vi "Run.vi"(2 "D_Angle":dbl, 3 "Angle":dbl, 4 "Encoder":dbl) -> (0 "PWM":dbl)   [LabVIEW 2018]
uses:
  Global_variables.vi
panel:
  out "exp(x)":dbl
  in  "Flag_Back 2":dbl
  in  "Count_keep_balance":dbl
  in  "Count_P2":dbl
  in  "count_position":dbl
  in  "Position_Max":dbl
  in  "Angle_Max":dbl
  in  "Count_Big_Angle":dbl
  in  "Flag_Back":dbl
  in  "Target_position":dbl
  in  "Count_Next":dbl
  in  "Count_FZ":dbl
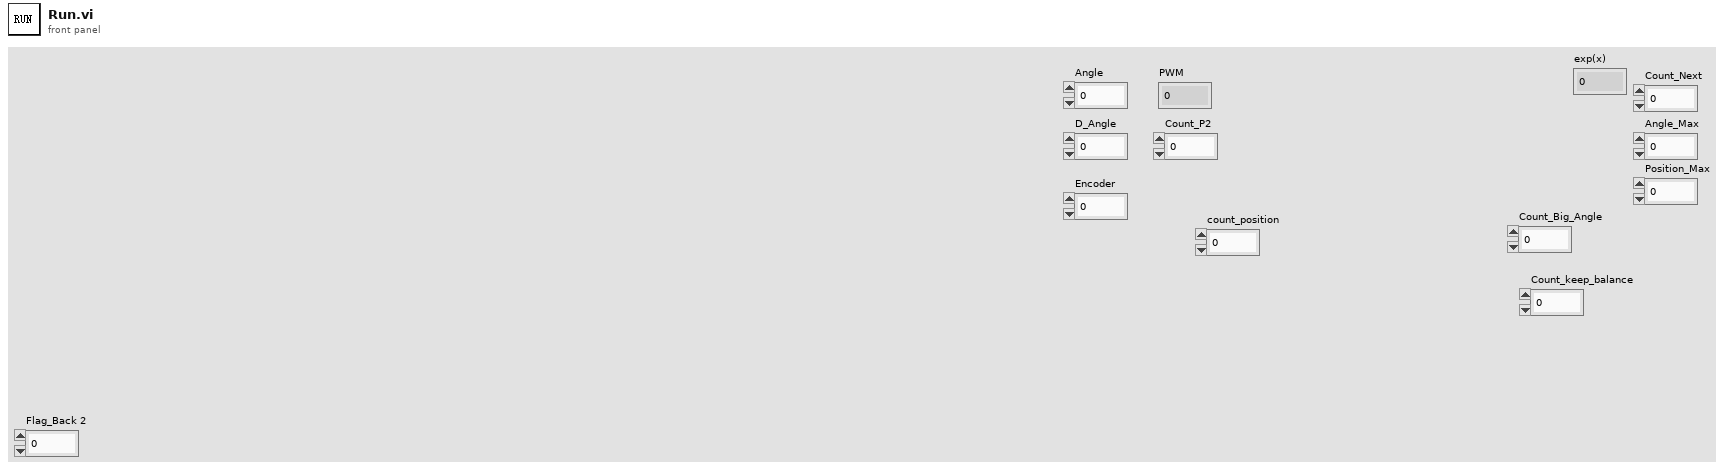
[diagram p1: front panel]
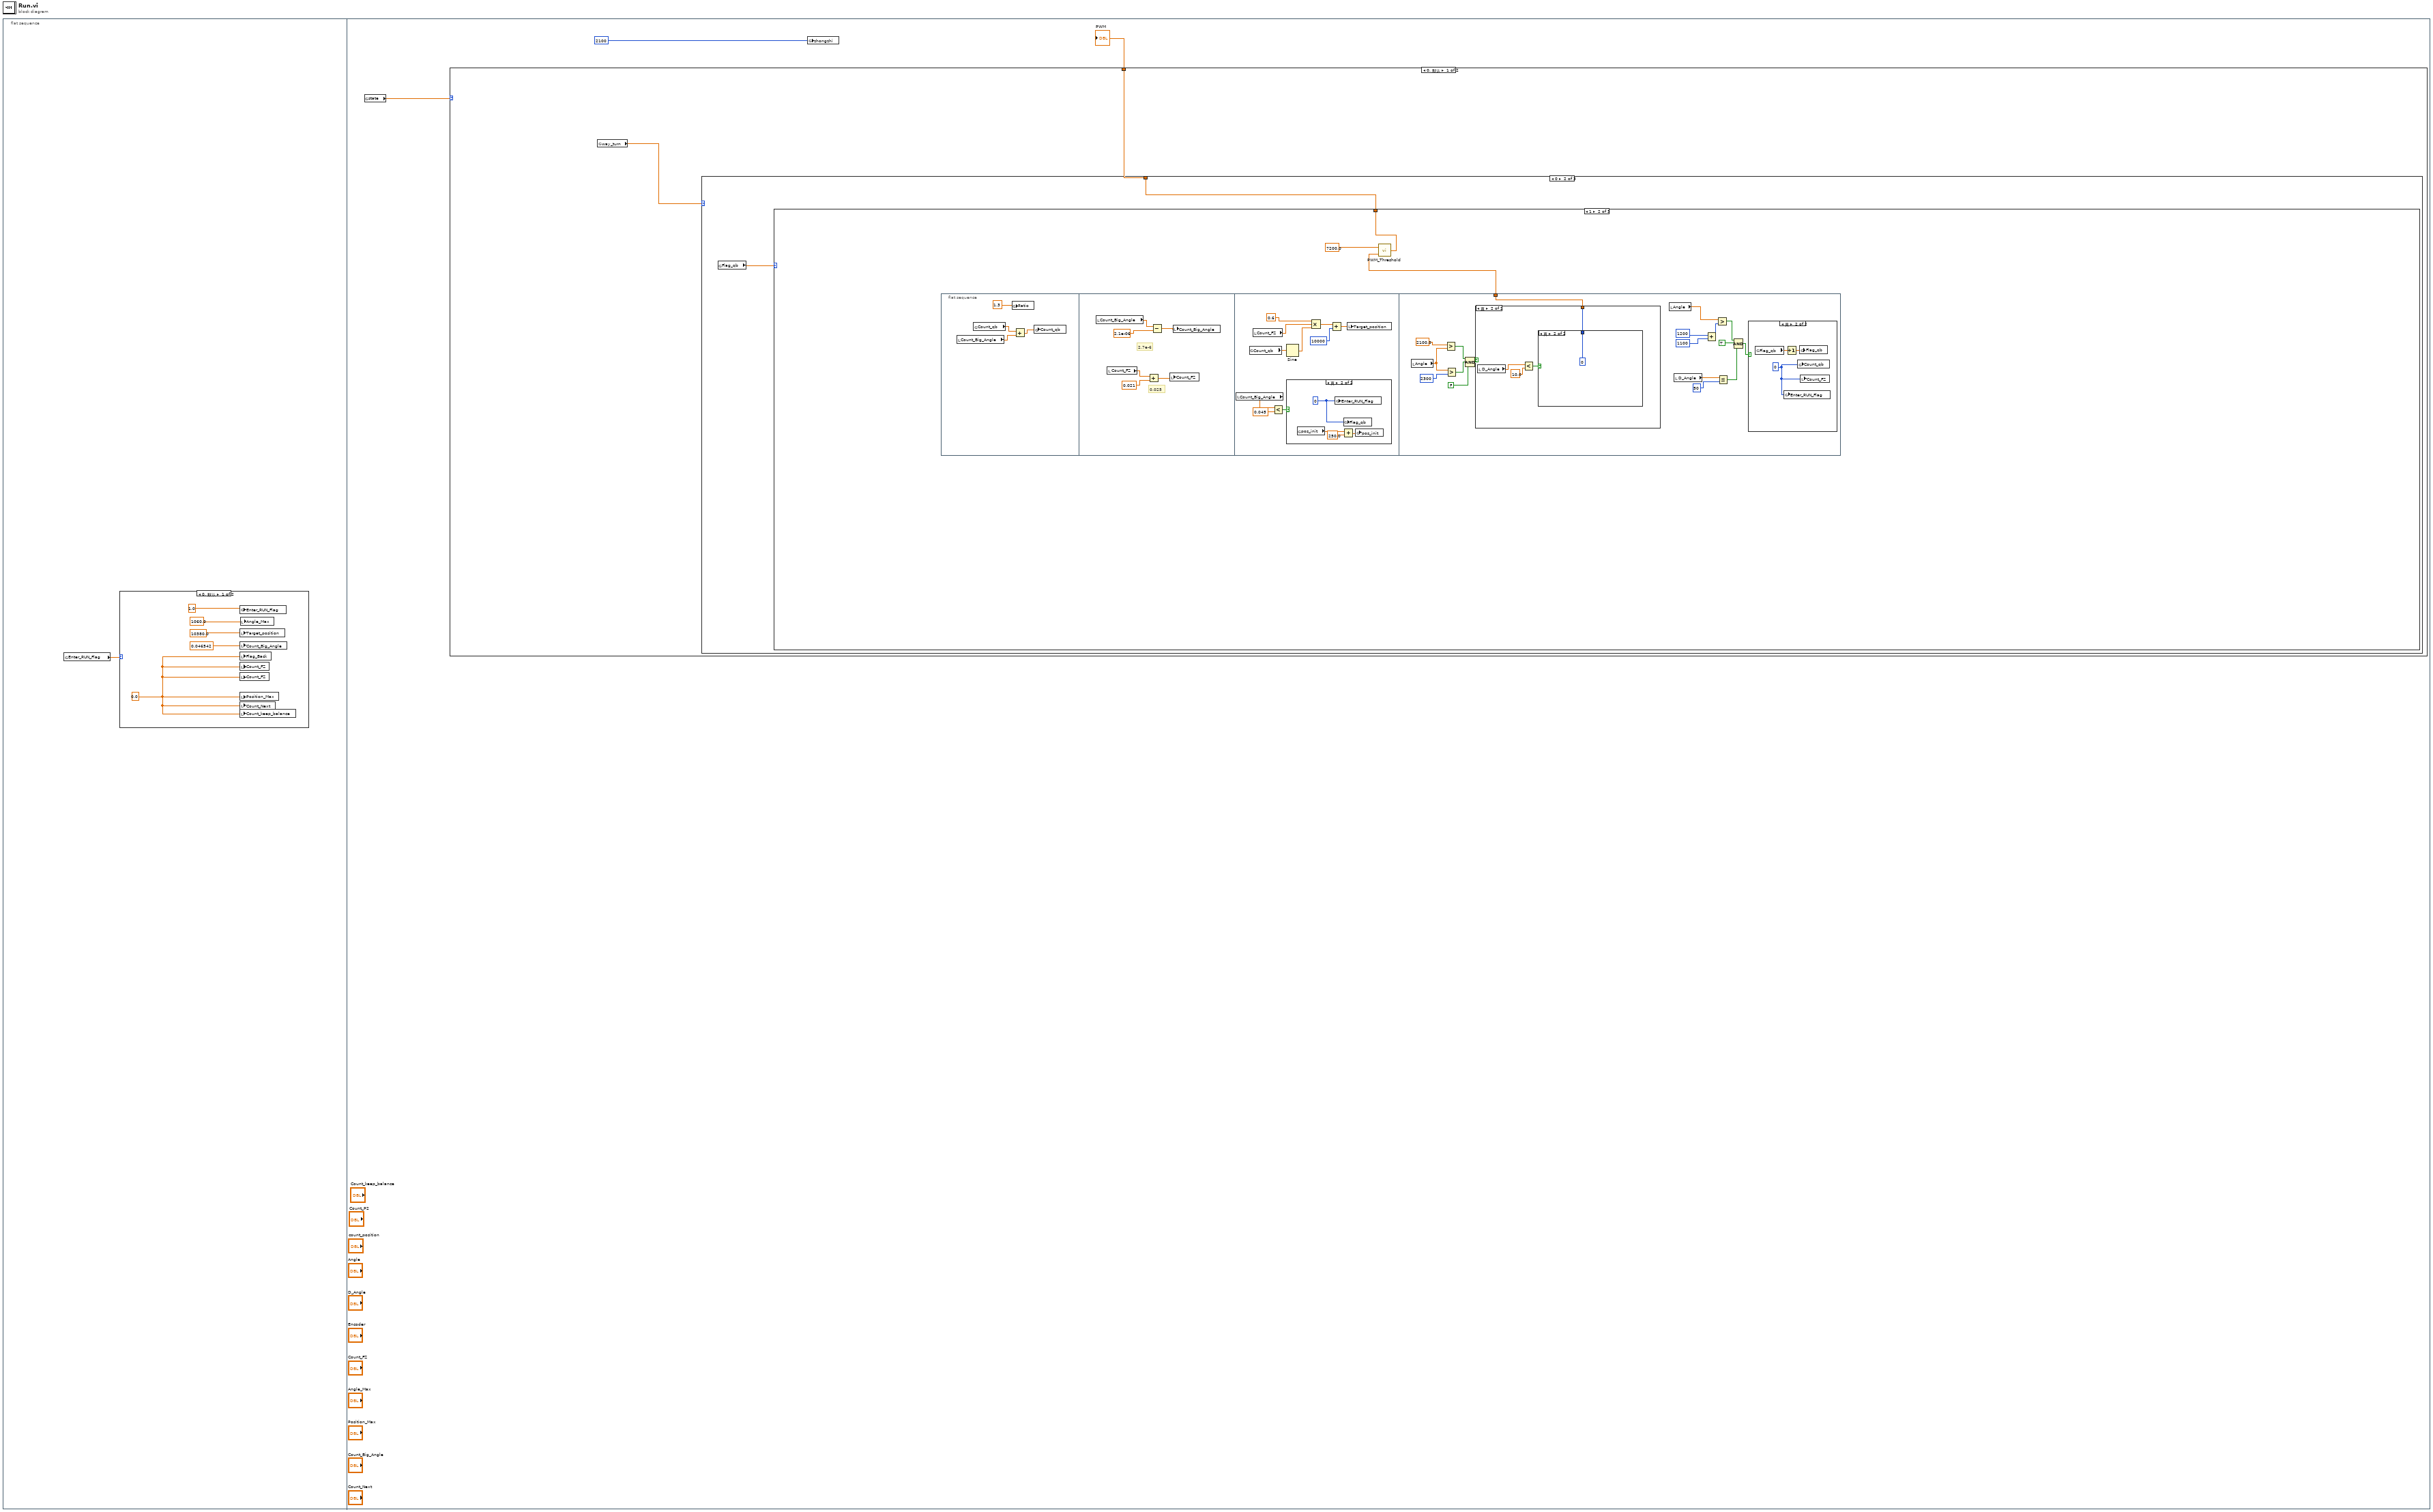
[diagram p0: block diagram]
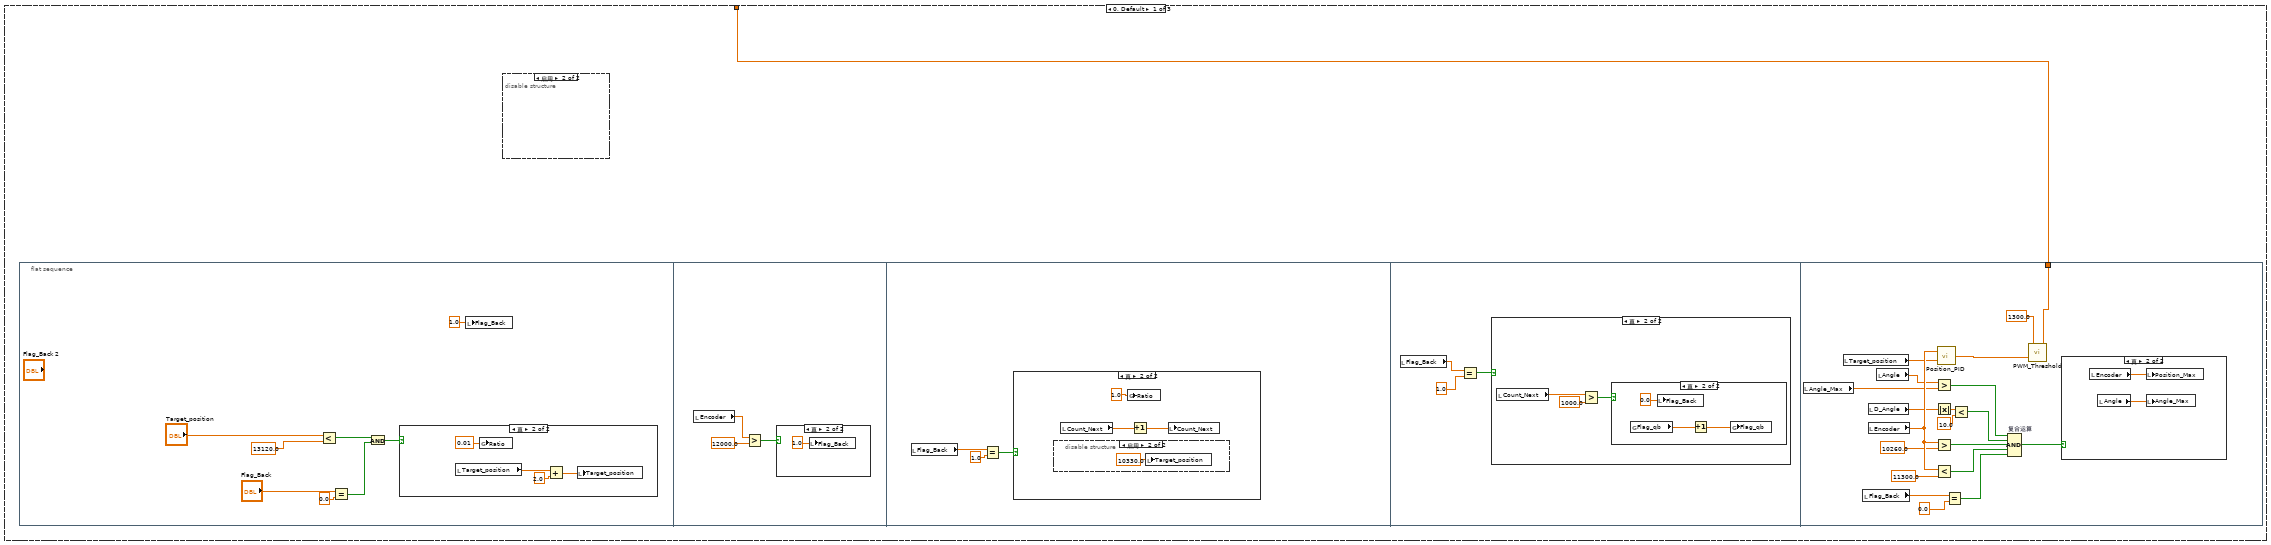
[diagram p4: hidden frame]
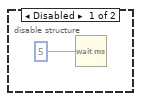
[diagram p5: hidden frame]
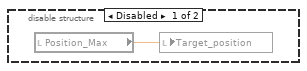
[diagram p9: hidden frame]
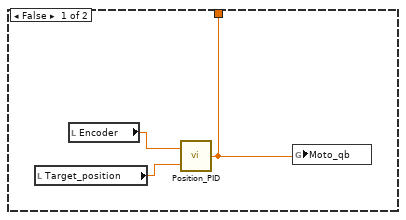
[diagram p14: hidden frame]
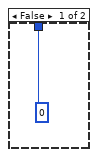
[diagram p15: hidden frame]
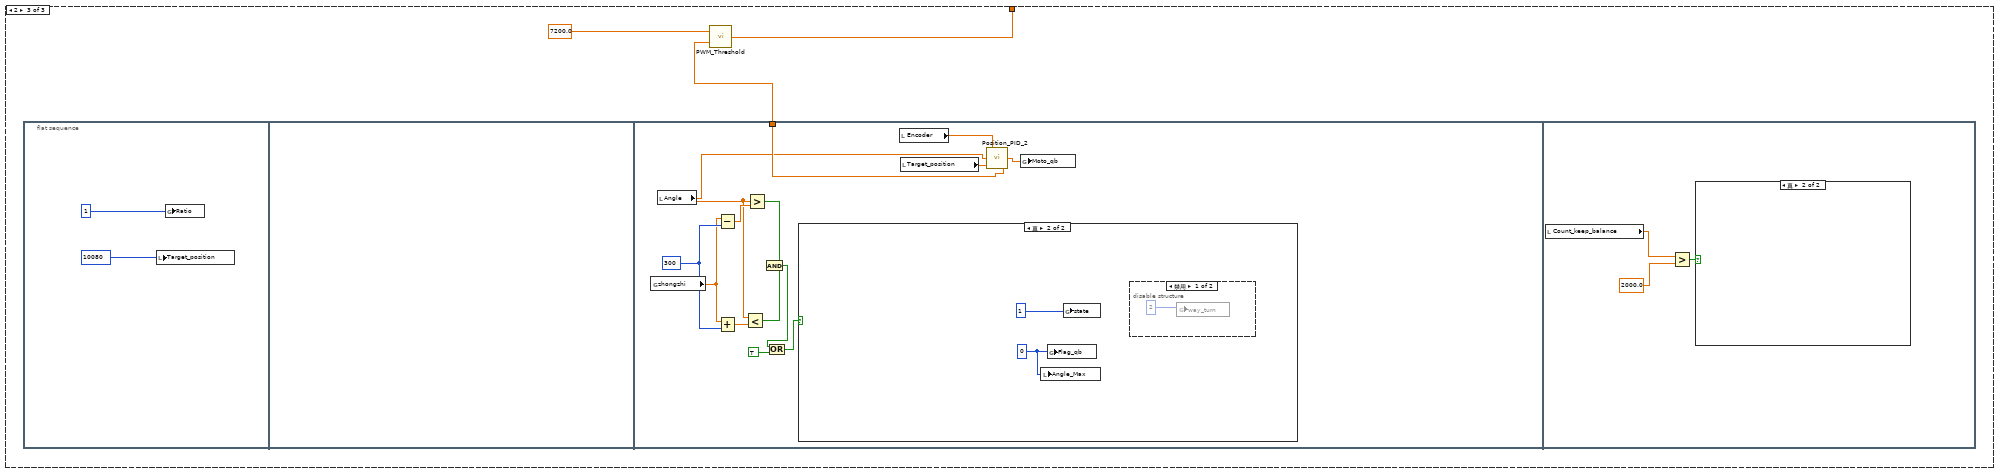
[diagram p17: hidden frame]
diagram:
  n1 = flat-sequence {
    frame #0 {
      n2 = global read "Global_variables.vi" "Enter_RUN_Flag"() -> (w1:dbl)
      n3 = case shown="0, 默认" w1 {
        frame 0, Default {
          w3 = 0.0 ("Position_Max")
          n4 = global write "Global_variables.vi" "Enter_RUN_Flag"(1.0 ("Enter_RUN_Flag")) -> ()
          n5 = local write "Target_position"(10380.0 ("Target_position")) -> ()
          n6 = local write "Count_Big_Angle"(0.046542 ("Count_Big_Angle")) -> ()
          n7 = local write "Flag_Back"(w3) -> ()
          n8 = local write "Count_FZ"(w3) -> ()
          n9 = local write "Count_FZ"(w3) -> ()
          n10 = local write "Position_Max"(w3) -> ()
          n11 = local write "Count_Next"(w3) -> ()
          n12 = local write "Count_keep_balance"(w3) -> ()
          n13 = local write "Angle_Max"(1060.0 ("Angle_Max")) -> ()
        }
        frame 1 {
        }
      }
    }
    frame #1 {
      n14 = global read "Global_variables.vi" "state"() -> (w8:dbl)
      n15 = case shown="0, 默认" w8 {
        tunnel: [w11 w162] -> w9
        frame 0, Default {
          n16 = global read "Global_variables.vi" "way_turn"() -> (w10:dbl)
          n17 = case shown="0" w10 {
            tunnel: [_ w12 _] -> w11
            frame 2, Default {
            }
            frame 0 {
              n18 = global read "Global_variables.vi" "Flag_qb"() -> (w13:dbl)
              n19 = case shown="1" w13 {
                tunnel: [w14 w73 w130] -> w12
                frame 0, Default {
                  n20 = flat-sequence {
                    tunnel: [w53] -> w14
                    frame #0 {
                      n21 = Less?(x="Target_position", y=13120.0) -> (x < y?=w20:bool)
                      n22 = Equal?(x="Flag_Back", y=0.0) -> (x = y?=w21:bool)
                      n23 = And(x=w20, y=w21) -> (x .and. y?=w23:bool)
                      n24 = case shown="真" w23 {
                        frame False {
                        }
                        frame True {
                          n25 = local read "Target_position"() -> (w27:dbl)
                          n26 = global write "Global_variables.vi" "Ratio"(0.01 ("Ratio")) -> ()
                          n27 = Add(x=w27, y=2.0) -> (x+y=w25:dbl)
                          n28 = local write "Target_position"(w25) -> ()
                        }
                      }
                      n29 = local write "Flag_Back"(1.0 ("Flag_Back")) -> ()
                    }
                    frame #1 {
                      n30 = local read "Encoder"() -> (w28:dbl)
                      n31 = Greater?(x=w28, y=12000.0) -> (0:w30:bool)
                      n32 = case shown="真" w30 {
                        frame False {
                        }
                        frame True {
                          n33 = local write "Flag_Back"(1.0 ("Flag_Back")) -> ()
                        }
                      }
                    }
                    frame #2 {
                      n34 = local read "Flag_Back"() -> (w34:dbl)
                      n35 = Equal?(x=w34, y=1.0) -> (x = y?=w33:bool)
                      n36 = case shown="真" w33 {
                        frame False {
                        }
                        frame True {
                          n37 = disable-structure shown="启用" {
                            frame Disabled {
                              n38 = local read "Position_Max"() -> (w38:dbl)
                              n39 = local write "Target_position"(w38) -> ()
                            }
                            frame Enabled {
                              n40 = local write "Target_position"(10330.0 ("Target_position")) -> ()
                            }
                          }
                          n41 = local read "Count_Next"() -> (w35:dbl)
                          n42 = global write "Global_variables.vi" "Ratio"(1.0 ("Ratio")) -> ()
                          n43 = Increment(x=w35) -> (x+1=w36:dbl)
                          n44 = local write "Count_Next"(w36) -> ()
                        }
                      }
                    }
                    frame #3 {
                      n45 = local read "Flag_Back"() -> (w42:dbl)
                      n46 = Equal?(x=w42, y=1.0) -> (x = y?=w40:bool)
                      n47 = case shown="真" w40 {
                        frame False {
                        }
                        frame True {
                          n48 = local read "Count_Next"() -> (w44:dbl)
                          n49 = Greater?(x=w44, y=1000.0) -> (0:w45:bool)
                          n50 = case shown="真" w45 {
                            frame False {
                            }
                            frame True {
                              n51 = global read "Global_variables.vi" "Flag_qb"() -> (w48:dbl)
                              n52 = local write "Flag_Back"(0.0 ("Flag_Back")) -> ()
                              n53 = Increment(x=w48) -> (x+1=w47:dbl)
                              n54 = global write "Global_variables.vi" "Flag_qb"(w47) -> ()
                            }
                          }
                        }
                      }
                    }
                    frame #4 {
                      n55 = local read "Angle_Max"() -> (w64:dbl)
                      n56 = local read "Target_position"() -> (w58:dbl)
                      n57 = local read "Flag_Back"() -> (w62:dbl)
                      n58 = local read "D_Angle"() -> (w52:dbl)
                      n59 = local read "Encoder"() -> (w67:dbl)
                      n60 = local read "Angle"() -> (w65:dbl)
                      n61 = Greater?(x=w65, y=w64) -> (0:w66:bool)
                      n62 = Absolute Value(x=w52) -> (abs(x)=w51:dbl)
                      n63 = Greater?(x=w67, y=10260.0) -> (0:w60:bool)
                      n64 = Less?(x=w67, y=11300.0) -> (x < y?=w61:bool)
                      n65 = call "Position_PID.vi"("Target_Position"=w58, "Encoder"=w67) -> ("PWM"=w59:dbl)
                      n66 = Equal?(x=w62, y=0.0) -> (x = y?=w63:bool)
                      n67 = Less?(x=w51, y=10.0) -> (x < y?=w49:bool)
                      n68 = Compound Arithmetic op=AND "复合运算"(w66, w49, w60, w61, w63) -> (w68:bool)
                      n69 = call "PWM_Threshold.vi"("Input_PWM"=w59, "Threshold"=1300.0) -> ("Trimmed_PWM"=w53:dbl)
                      n70 = case shown="真" w68 {
                        frame False {
                        }
                        frame True {
                          n71 = local read "Encoder"() -> (w69:dbl)
                          n72 = local read "Angle"() -> (w70:dbl)
                          n73 = local write "Position_Max"(w69) -> ()
                          n74 = local write "Angle_Max"(w70) -> ()
                        }
                      }
                    }
                  }
                  n75 = disable-structure shown="启用" {
                    frame Disabled {
                      n76 = Wait (ms)(milliseconds to wait=u32 5 ("等待时间（毫秒）")) -> ()  [unwired: 1 out]
                    }
                    frame Enabled {
                    }
                  }
                }
                frame 1 {
                  n77 = flat-sequence {
                    tunnel: [w99] -> w72
                    frame #0 {
                      n78 = local read "Count_Big_Angle"() -> (w74:dbl)
                      n79 = global read "Global_variables.vi" "Count_qb"() -> (w75:dbl)
                      n80 = global write "Global_variables.vi" "Ratio"(1.3) -> ()
                      n81 = Add(x=w75, y=w74) -> (x+y=w76:dbl)
                      n82 = global write "Global_variables.vi" "Count_qb"(w76) -> ()
                    }
                    frame #1 {
                      # "2.7e-6"
                      # "0.025"
                      n83 = local read "Count_Big_Angle"() -> (w83:dbl)
                      n84 = local read "Count_FZ"() -> (w80:dbl)
                      n85 = Add(x=w80, y=0.021) -> (x+y=w78:dbl)
                      n86 = Subtract(x=w83, y=2.1e-06) -> (x-y=w81:dbl)
                      n87 = local write "Count_FZ"(w78) -> ()
                      n88 = local write "Count_Big_Angle"(w81) -> ()
                    }
                    frame #2 {
                      n89 = local read "Count_Big_Angle"() -> (w85:dbl)
                      n90 = global read "Global_variables.vi" "Count_qb"() -> (w91:dbl)
                      n91 = local read "Count_FZ"() -> (w92:dbl)
                      n92 = Less?(x=w85, y=0.045) -> (x < y?=w86:bool)
                      n93 = Sine(x=w91) -> (sin(x)=w90:dbl)
                      n94 = case shown="真" w86 {
                        frame False {
                        }
                        frame True {
                          w97 = 0
                          n95 = global read "Global_variables.vi" "pos_init"() -> (w94:dbl)
                          n96 = global write "Global_variables.vi" "Enter_RUN_Flag"(w97) -> ()
                          n97 = Add(x=w94, y=250.0) -> (x+y=w96:dbl)
                          n98 = global write "Global_variables.vi" "Flag_qb"(w97) -> ()
                          n99 = global write "Global_variables.vi" "pos_init"(w96) -> ()
                        }
                      }
                      n100 = Compound Arithmetic op=MULTIPLY(0.6, w92, w90) -> (w88:dbl)
                      n101 = Add(x=w88, y=10000) -> (x+y=w89:dbl)
                      n102 = local write "Target_position"(w89) -> ()
                    }
                    frame #3 {
                      n103 = local read "Angle"() -> (w104:dbl)
                      n104 = Greater?(x=2100.0 ("y"), y=w104) -> (0:w101:bool)
                      n105 = Greater?(x=w104, y=2300) -> (0:w100:bool)
                      n106 = Compound Arithmetic op=AND ("复合运算")(w101, w100, FALSE) -> (w102:bool)
                      n107 = case shown="真" w102 {
                        tunnel: [w116 w122] -> w99
                        frame False {
                          n108 = local read "Target_position"() -> (w118:dbl)
                          n109 = local read "Encoder"() -> (w117:dbl)
                          n110 = call "Position_PID.vi"("Target_Position"=w118, "Encoder"=w117) -> ("PWM"=w116:dbl)
                          n111 = global write "Global_variables.vi" "Moto_qb"(w116) -> ()
                        }
                        frame True {
                          n112 = local read "D_Angle"() -> (w121:dbl)
                          n113 = Less?(x=w121, y=10.0) -> (x < y?=w119:bool)
                          n114 = case shown="真" w119 {
                            tunnel: [0 0] -> w122
                            frame False {
                            }
                            frame True {
                            }
                          }
                        }
                      }
                      n115 = local read "Angle"() -> (w108:dbl)
                      n116 = local read "D_Angle"() -> (w113:dbl)
                      n117 = Add(x=1200, y=1100) -> (x+y=w115:i32)
                      n118 = Greater?(x=w108, y=w115) -> (0:w111:bool)
                      n119 = Less Or Equal?(x=w113, y=50) -> (x <= y?=w110:bool)
                      n120 = Compound Arithmetic op=AND ("复合运算")(w111, TRUE, w110) -> (w109:bool)
                      n121 = case shown="真" w109 {
                        frame False {
                        }
                        frame True {
                          w125 = 0
                          n122 = global read "Global_variables.vi" "Flag_qb"() -> (w127:dbl)
                          n123 = global write "Global_variables.vi" "Enter_RUN_Flag"(w125) -> ()
                          n124 = Increment(x=w127) -> (x+1=w126:dbl)
                          n125 = global write "Global_variables.vi" "Count_qb"(w125) -> ()
                          n126 = global write "Global_variables.vi" "Flag_qb"(w126) -> ()
                          n127 = local write "Count_FZ"(w125) -> ()
                        }
                      }
                    }
                  }
                  n128 = call "PWM_Threshold.vi"("Input_PWM"=w72, "Threshold"=7200.0) -> ("Trimmed_PWM"=w73:dbl)
                }
                frame 2 {
                  n129 = flat-sequence {
                    tunnel: [w139] -> w129
                    frame #0 {
                      n130 = local write "Target_position"(10080) -> ()
                      n131 = global write "Global_variables.vi" "Ratio"(1) -> ()
                    }
                    frame #1 {
                    }
                    frame #2 {
                      w141 = 300
                      n132 = global read "Global_variables.vi" "zhongzhi"() -> (w140:dbl)
                      n133 = local read "Angle"() -> (w136:dbl)
                      n134 = Subtract(x=w140, y=w141) -> (x-y=w142:dbl)
                      n135 = Add(x=w140, y=w141) -> (x+y=w145:dbl)
                      n136 = Less?(x=w136, y=w145) -> (x < y?=w143:bool)
                      n137 = Greater?(x=w136, y=w142) -> (0:w144:bool)
                      n138 = And(x=w144, y=w143) -> (x .and. y?=w134:bool)
                      n139 = Or(x=w134, y=TRUE) -> (x .or. y?=w135:bool)
                      n140 = case shown="真" w135 {
                        frame False {
                        }
                        frame True {
                          w147 = 0
                          n141 = local write "Angle_Max"(w147) -> ()
                          n142 = global write "Global_variables.vi" "Flag_qb"(w147) -> ()
                          n143 = global write "Global_variables.vi" "state"(1) -> ()
                          n144 = disable-structure shown="禁用" {
                            frame Disabled {
                              n145 = global write "Global_variables.vi" "way_turn"(2) -> ()
                            }
                            frame Enabled {
                            }
                          }
                        }
                      }
                      n146 = local read "Encoder"() -> (w138:dbl)
                      n147 = local read "Target_position"() -> (w137:dbl)
                      n148 = call "Position_PID_2.vi"("Target_Position"=w137, "Angle"=w136, "Encoder"=w138) -> ("PWM"=w139:dbl)
                      n149 = global write "Global_variables.vi" "Moto_qb"(w139) -> ()
                    }
                    frame #3 {
                      n150 = local read "Count_keep_balance"() -> (w150:dbl)
                      n151 = Greater?(x=w150, y=2000.0) -> (0:w151:bool)
                      n152 = case shown="真" w151 {
                        frame False {
                        }
                        frame True {
                        }
                      }
                    }
                  }
                  n153 = call "PWM_Threshold.vi"("Input_PWM"=w129, "Threshold"=7200.0) -> ("Trimmed_PWM"=w130:dbl)
                }
              }
            }
            frame 1 {
              w159 = 200
              n154 = global read "Global_variables.vi" "zhongzhi"() -> (w158:dbl)
              n155 = local read "Angle"() -> (w155:dbl)
              n156 = Subtract(x=w158, y=w159) -> (x-y=w156:dbl)
              n157 = Add(x=w158, y=w159) -> (x+y=w157:dbl)
              n158 = Less?(x=w155, y=w157) -> (x < y?=w154:bool)
              n159 = Greater?(x=w155, y=w156) -> (0:w153:bool)
              n160 = And(x=w154, y=w153) -> (x .and. y?=w152:bool)
              n161 = case shown="假" w152 {
                frame False {
                }
                frame True {
                  n162 = global write "Global_variables.vi" "way_turn"(2) -> ()
                  n163 = global write "Global_variables.vi" "state"(1) -> ()
                }
              }
            }
          }
        }
        frame 1 {
          n164 = flat-sequence {
            tunnel: [w201] -> w162
            frame #0 {
              # "244"
              n165 = local read "Count_keep_balance"() -> (w163:dbl)
              n166 = local read "Angle"() -> (w168:dbl)
              n167 = Increment(x=w163) -> (x+1=w164:dbl)
              n168 = call "Balance_PWM.vi"("Balance_Ratio"=0, "Balance_KD"=244, "Balance_KP"=50, "Angle"=w168) -> ("Balance_PWM"=w169:dbl)
              n169 = local write "Count_keep_balance"(w164) -> ()
              n170 = global write "Global_variables.vi" "Balance_PWM"(w169) -> ()
            }
            frame #1 {
              n171 = global read "Global_variables.vi" "Flag_qb 2"() -> (w170:dbl)
              n172 = case shown="1" w170 {
                frame 0, Default {
                  n173 = flat-sequence {
                    frame #0 {
                      w171 = 200
                      n174 = local read "Angle"() -> (w174:dbl)
                      n175 = global read "Global_variables.vi" "zhongzhi"() -> (w172:dbl)
                      n176 = Add(x=w172, y=w171) -> (x+y=w175:dbl)
                      n177 = Subtract(x=w172, y=w171) -> (x-y=w173:dbl)
                      n178 = Less?(x=w174, y=w175) -> (x < y?=w178:bool)
                      n179 = Greater?(x=w174, y=w173) -> (0:w177:bool)
                      n180 = And(x=w177, y=w178) -> (x .and. y?=w176:bool)
                      n181 = case shown="真" w176 {
                        frame False {
                        }
                        frame True {
                          n182 = local read "count_position"() -> (w180:dbl)
                          n183 = Increment(x=w180) -> (x+1=w179:dbl)
                          n184 = local write "count_position"(w179) -> ()
                        }
                      }
                    }
                    frame #1 {
                      n185 = local read "count_position"() -> (w182:dbl)
                      n186 = Greater?(x=w182, y=60) -> (0:w183:bool)
                      n187 = case shown="真" w183 {
                        frame False {
                        }
                        frame True {
                          n188 = local write "count_position"(0) -> ()
                          n189 = global write "Global_variables.vi" "Flag_qb 2"(1) -> ()
                        }
                      }
                    }
                  }
                }
                frame 1 {
                  n190 = local read "Count_P2"() -> (w189:dbl)
                  n191 = Increment(x=w189) -> (x+1=w188:dbl)
                  n192 = local write "Count_P2"(w188) -> ()
                  n193 = Greater?(x=w188, y=4) -> (0:w186:bool)
                  n194 = case shown="真" w186 {
                    frame False {
                    }
                    frame True {
                      n195 = local read "Encoder"() -> (w194:dbl)
                      n196 = local write "Count_P2"(0) -> ()
                      n197 = call "Postion_PWM.vi"("Position_KD"=600, "Position_KP"=25, "Encoder"=w194) -> ("Postion_PWM"=w193:dbl)
                      n198 = global write "Global_variables.vi" "Position_PWM"(w193) -> ()
                    }
                  }
                }
              }
            }
            frame #2 {
              n199 = local read "Count_keep_balance"() -> (w203:dbl)
              n200 = global read "Global_variables.vi" "zhongzhi"() -> (w209:dbl)
              n201 = local read "Angle"() -> (w208:dbl)
              n202 = Multiply(x=w203, y=-0.002) -> (x*y=w204:dbl)
              n203 = global read "Global_variables.vi" "Balance_PWM"() -> (w200:dbl)
              n204 = global read "Global_variables.vi" "Position_PWM"() -> (w206:dbl)
              n205 = Subtract(x=w208, y=w209) -> (x-y=w210:dbl)
              n206 = Exponential(1:w204) -> (0:w197:dbl)
              n207 = Absolute Value(x=w210) -> (abs(x)=w211:dbl)
              n208 = Multiply(x=2.0, y=w197) -> (x*y=w198:dbl)
              n209 = Greater?(x=w211, y=800.0) -> (0:w212:bool)
              n210 = Increment(x=w198) -> (x+1=w195:dbl)
              "exp(x)" <- w195
              n211 = Multiply(x=w200, y=w195) -> (x*y=w199:dbl)
              n212 = call "Generate_PWM.vi"("Balance_PWM"=w199, "Position_PWM"=w206) -> ("PWM"=w205:dbl)
              n213 = case shown="真" w212 {
                tunnel: w205 -> [w213 w219]
                tunnel: [w213 w217] -> w201
                frame False {
                }
                frame True {
                  n214 = global read "Global_variables.vi" "way_turn"() -> (w215:dbl)
                  n215 = Equal?(x=w215, y=0) -> (x = y?=w216:bool)
                  n216 = case shown="真" w216 {
                    frame False {
                    }
                    frame True {
                      n217 = global read "Global_variables.vi" "pos_init"() -> (w222:dbl)
                      n218 = global write "Global_variables.vi" "Flag_qb"(0) -> ()
                      n219 = global write "Global_variables.vi" "state"(0.0 ("state")) -> ()
                      n220 = Add(x=w222, y=250.0) -> (x+y=w223:dbl)
                      n221 = local write "Count_keep_balance"(0.0 ("Count_keep_balance")) -> ()
                      n222 = global write "Global_variables.vi" "pos_init"(w223) -> ()
                    }
                  }
                  n223 = Multiply(x=w219, y=0.0) -> (x*y=w217:dbl)
                }
              }
            }
          }
        }
      }
      "PWM" <- w9
      n224 = global write "Global_variables.vi" "zhongzhi"(2100) -> ()
    }
  }
